vi "Handle Drag Starting.vi"(4 "Mods":cluster{"Double Click":bool, "Menu Key":bool}, 5 "Drag Mode":enum32{"copy or move", "copy only", "move only"}(ring), 6 "PlatMods":T3, 7 "Button":u16, 8 "error in (no error)":errorcluster, 9 "Coords":T2, 10 "Data":T4(array[cluster]), 11 "Test Executive Builder View in":refnum<class "Test Executive Builder View.lvclass">) -> (0 "error out":errorcluster, 2 "Drag Starting Filtered Event Data":T1, 3 "Test Executive Builder View out":refnum<class "Test Executive Builder View.lvclass">)   [LabVIEW 2017, in "Test Executive Builder View.lvclass"]
uses:
  <vilib>/gpm_packages/@cs/Test-executive-builder/Source/Test Executive Builder View/Test Executive Builder View/Test Executive Builder View.lvclass
  <vilib>/Utility/miscctls.llb/LVPoint32TypeDef.ctl
  <vilib>/gpm_packages/@cs/Test-executive-builder/Source/Application Dependencies/Drag Starting Filtered Event Data.ctl
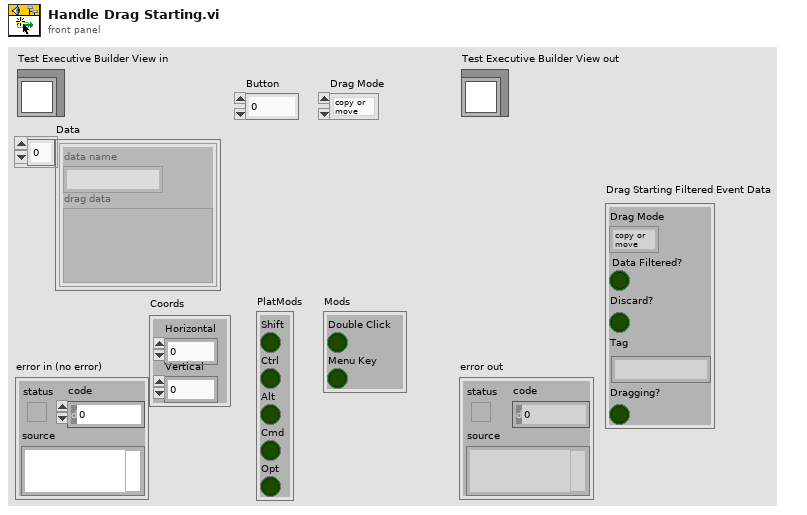
[diagram p1: front panel]
types:
  T1 = typedef "Drag Starting Filtered Event Data.ctl" = cluster{"Drag Mode":enum32{"copy or move", "copy only", "move only"}, "Data Filtered?":bool, "Discard?":bool, "Tag":string, "Dragging?":bool}
  T2 = typedef "LVPoint32TypeDef.ctl" = cluster{"Horizontal":i32, "Vertical":i32}
  T3 = cluster{"Shift":bool, "Ctrl":bool, "Alt":bool, "Cmd":bool, "Opt":bool}
  T4 = cluster{"data name":string, "drag data":variant}[]
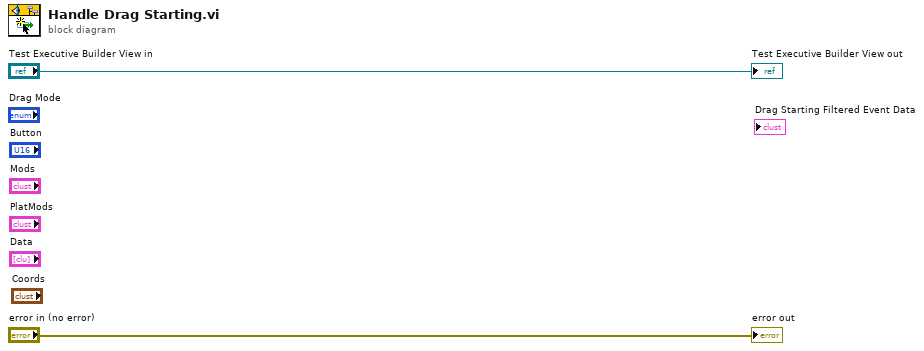
[diagram p0: block diagram]
diagram:
  "error out" <- "error in (no error)"
  "Test Executive Builder View out" <- "Test Executive Builder View in"
